vi "picoExtractSettings.vi"(11 "Rapid Block Acquisition Settings":T1) -> (1 "Down-Sample Mode":i32, 2 "Down Sample Ratio":u32, 3 "Numeric":i32)   [LabVIEW 2011]
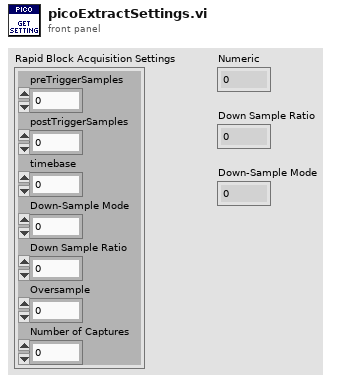
[diagram p1: front panel]
types:
  T1 = cluster{"preTriggerSamples":u32, "postTriggerSamples":u32, "timebase":u32, "Down-Sample Mode":i32, "Down Sample Ratio":u32, "Oversample":i16, "Number of Captures":u32}
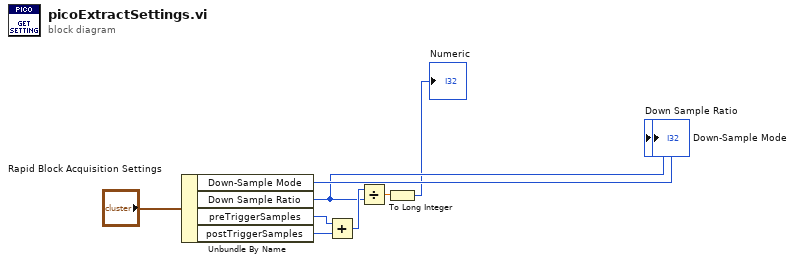
[diagram p0: block diagram]
diagram:
  n1 = Unbundle By Name("Rapid Block Acquisition Settings") -> ("Down-Sample Mode"=→"Down-Sample Mode":i32, "Down Sample Ratio"=w6:u32, "preTriggerSamples"=w1:u32, "postTriggerSamples"=w3:u32)
  "Down Sample Ratio" <- w6
  n2 = Add(x=w1, y=w3) -> (x+y=w8:u32)
  n3 = Divide(x=w8, y=w6) -> (x/y=w4:dbl)
  n4 = To Long Integer(number=w4) -> (32bit integer=→"Numeric":i32)
